vi "GetFrameRate.vi"(8 "error in (no error)":errorcluster, 11 "CameraTestingBL in":refnum<class "CameraTesting.lvclass">) -> (0 "error out":errorcluster, 3 "CameraTestingBL out":refnum<class "CameraTesting.lvclass">)   [LabVIEW 2020, in "CameraTesting.lvlib" / "CameraTesting.lvclass"]
doc: "Get the frame rate of the camera"
uses:
  CameraTesting.lvclass
  CameraTesting.lvclass/CameraTesting.ctl
  Camera/ICamera/ICamera/ICamera.lvclass
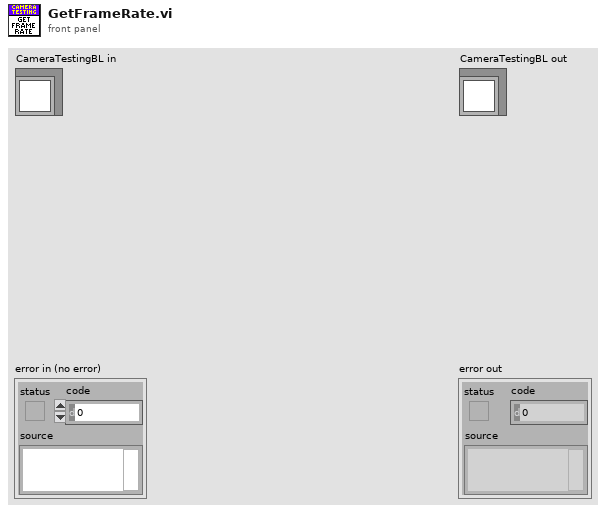
[diagram p1: front panel]
types:
  T1 = typedef "ICameraTesting.lvlib/ICameraTesting.lvclass/FrameRateValReceived.ctl" = refnum<user-event>
  T2 = typedef "ICameraTesting.lvlib/ICameraTesting.lvclass/StatusUpdated.ctl" = refnum<user-event>
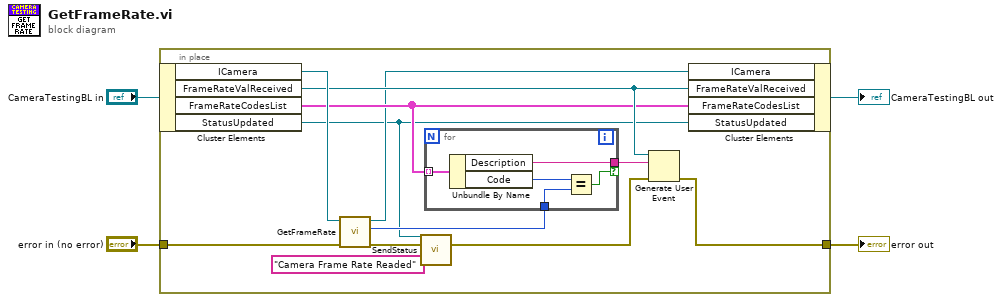
[diagram p0: block diagram]
diagram:
  n1 = in-place {
    in-place-border: "error in (no error)" -> [w16]
    in-place-border: [w13] -> w3
    n2 = in-place-cluster #1("CameraTestingBL in") -> ("ICamera"=w15:refnum<class "ICamera.lvclass">, "FrameRateValReceived"=w14:T1, "FrameRateCodesList"=w12:cluster{"Description":string, "Code":u8}[], "StatusUpdated"=w5:T2)
    n3 = call-dynamic "GetFrameRate.vi"("error in (no error)"=w16, "ICamera in"=w15) -> ("error out"=w7:errorcluster, "Frame Rate"=w11:u8, "ICamera out"=w9:refnum<class "ICamera.lvclass">)  [unwired: 7 in]
    n4 = call "SendStatus.vi"("StatusUsrEvn"=w5, "error in"=w7, "Text"="Camera Frame Rate Readed") -> ("error out"=w6:errorcluster)  [unwired: 24 in]
    n5 = for {
      tunnel: w12 -> [w21] mode=indexing
      tunnel: [w20] -> w10 if=w18
      tunnel: w11 -> [w17]
      n6 = Unbundle By Name(w21) -> ("Description"=w20:string, "Code"=w19:u8)
      n7 = Equal?(x=w19, y=w17) -> (x = y?=w18:bool)
    }
    n8 = Generate User Event(user event=w14, event data cluster=w10, error in=w6) -> (error out=w13:errorcluster)  [unwired: 1 in, 1 out]
    n9 = in-place-cluster #1("ICamera"=w9, "FrameRateValReceived"=w14, "FrameRateCodesList"=w12, "StatusUpdated"=w5) -> (→"CameraTestingBL out":refnum<class "CameraTesting.lvclass">)
  }
  "error out" <- w3
